vi "Flags to Item Symbols.vi"(11 "Flags":bool[](array[boolean])) -> (3 "Item Symbols":i32[](array[numeric]))   [LabVIEW 2020, in "UIM.lvlib" / "UIM.lvclass"]
uses:
  UIM.lvclass
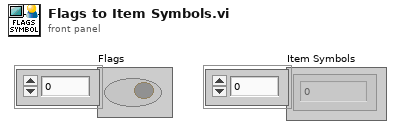
[diagram p1: front panel]
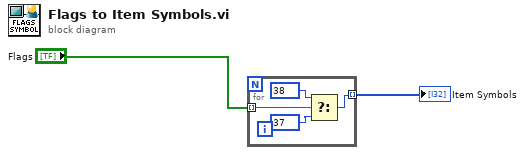
[diagram p0: block diagram]
diagram:
  n1 = for {
    tunnel: "Flags" -> [w6] mode=indexing
    tunnel: [w3] -> w2 mode=indexing
    n2 = Select(t=38, s=w6, f=37) -> (s? t:f=w3:i32)
  }
  "Item Symbols" <- w2
